vi "SendCommand.vi"(8 "error in (no error)":errorcluster, 10 "Command":string, 11 "VISA resource name":refnum<visa-resource-name>) -> (0 "error out":errorcluster, 3 "VISA resource name out":refnum<visa-resource-name>)   [LabVIEW 2019]
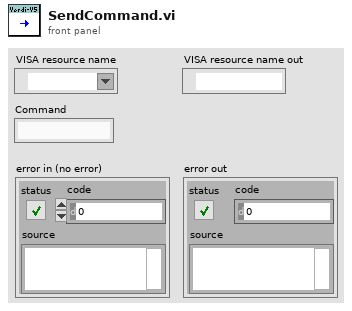
[diagram p1: front panel]
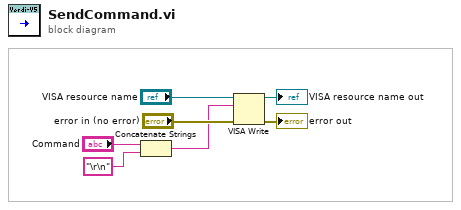
[diagram p0: block diagram]
diagram:
  n1 = Concatenate Strings("Command", "\r\n" ("string")) -> (w3:string)
  n2 = VISA Write(VISA resource name="VISA resource name", write buffer=w3, error in (no error)="error in (no error)") -> (VISA resource name out=→"VISA resource name out":refnum<visa-resource-name>, error out=→"error out":errorcluster)  [unwired: 1 out]
